vi "NIST Read Binary Data.vi"(0 "Wave File Path IN":path, 5 "error in (no error)":errorcluster, 6 "NIST File Header":T1) -> (14 "Wave File Path OUT":path, 16 "Data":waveform(dbl)[](array[waveform]), 19 "error out":errorcluster)   [LabVIEW 2022 SP3, in "WaveFile.lvclass"]
uses:
  WaveFile.lvclass
  utils/NIST File Header.ctl
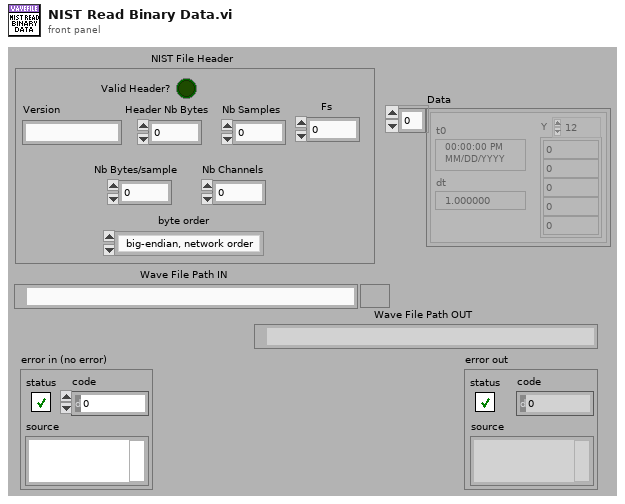
[diagram p1: front panel]
types:
  T1 = typedef "WaveFile.lvclass/NIST File Header.ctl" = cluster{"Version":string, "Header Nb Bytes":i32, "Nb Samples":i32, "Nb Bytes/sample":i32, "Nb Channels":i32, "byte order":enum16{"big-endian, network order", "native, host order", "little-endian"}, "Fs":dbl, "Valid Header?":bool}
  T2 = enum16{"big-endian, network order", "native, host order", "little-endian"}
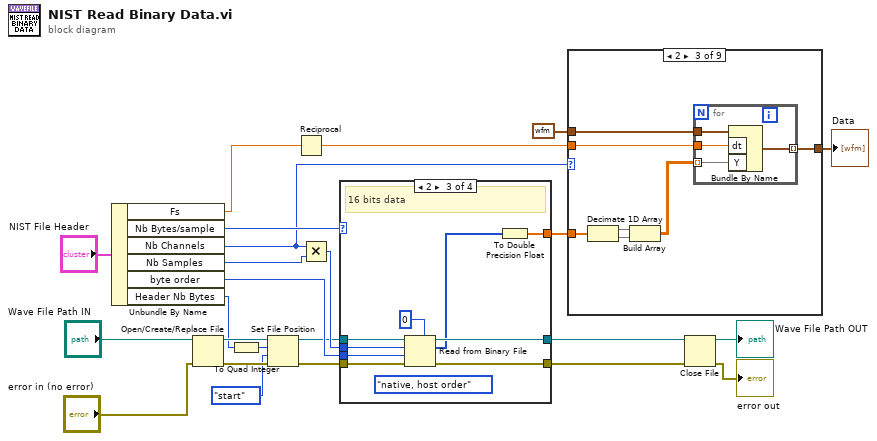
[diagram p0: block diagram]
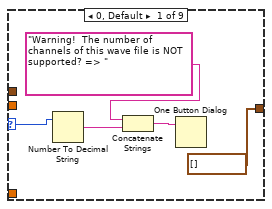
[diagram p2: hidden frame]
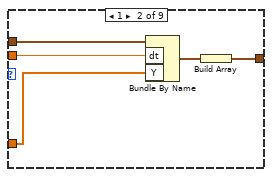
[diagram p3: hidden frame]
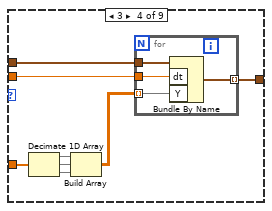
[diagram p4: hidden frame]
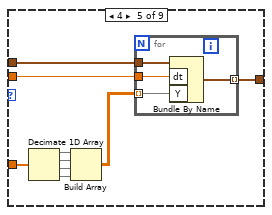
[diagram p5: hidden frame]
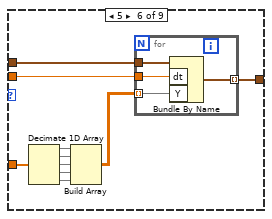
[diagram p6: hidden frame]
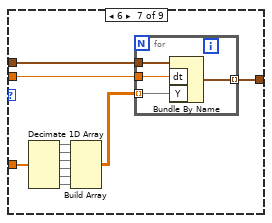
[diagram p7: hidden frame]
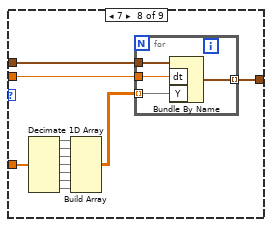
[diagram p8: hidden frame]
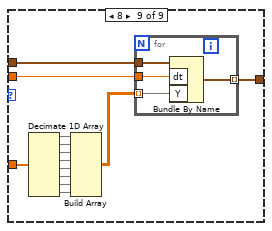
[diagram p9: hidden frame]
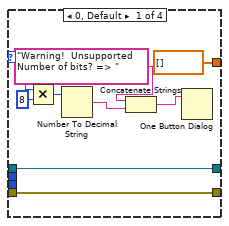
[diagram p10: hidden frame]
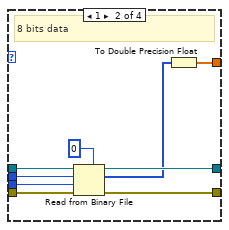
[diagram p11: hidden frame]
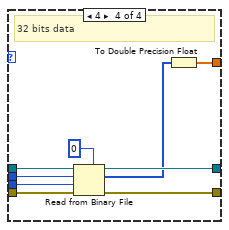
[diagram p12: hidden frame]
diagram:
  n1 = Unbundle By Name("NIST File Header") -> ("Fs"=w14:dbl, "Nb Bytes/sample"=w18:i32, "Nb Channels"=w15:i32, "Nb Samples"=w17:i32, "byte order"=w23:T2, "Header Nb Bytes"=w3:i32)
  n2 = Open/Create/Replace File(file path (use dialog)="Wave File Path IN", error in="error in (no error)") -> (refnum out=w7:refnum<file>, error out=w4:errorcluster)  [unwired: 4 in, 1 out]
  n3 = To Quad Integer(1:w3) -> (0:w2:i64)
  n4 = Set File Position(offset (in bytes) (0)=w2, refnum=w7, from (0:start)=enum16{"start", "end", "current"}."start", error in=w4) -> (refnum out=w6:refnum<file>, error out=w5:errorcluster)
  n5 = Reciprocal(x=w14) -> (1/x=w13:dbl)
  n6 = Multiply(x=w15, y=w17) -> (x*y=w16:i32)
  n7 = case shown="2" w18 {
    selector: w18 -> [w30 _ _ _]
    tunnel: w6 -> [w32 w42 w51 w60]
    tunnel: w5 -> [w31 w41 w50 w59]
    tunnel: w23 -> [_ w34 w43 w58]
    tunnel: w16 -> [_ w40 w49 w57]
    tunnel: [w32 w39 w48 w56] -> w20
    tunnel: [w31 w38 w47 w55] -> w19
    tunnel: [dbl[] [] w35 w44 w52] -> w11
    frame 0, Default {
      n8 = Multiply(x=w30, y=8) -> (x*y=w28:i32)
      n9 = Number To Decimal String(number=w28) -> (decimal integer string=w26:string)  [unwired: 1 in]
      n10 = Concatenate Strings("Warning!  Unsupported Number of bits? => " ("message"), w26) -> (w25:string)
      n11 = One Button Dialog(message=w25) -> ()  [unwired: 1 in, 1 out]
    }
    frame 1 {
      # "8 bits data"
      n12 = Read from Binary File(5:i8 0, 8:w41, 9:w34, 10:w40, 11:w42) -> (0:w38:errorcluster, 2:w36:i8[], 3:w39:refnum<file>)  [unwired: 1 in, 1 out]
      n13 = To Double Precision Float(number=w36) -> (double precision float=w35:dbl[])
    }
    frame 2 {
      (unwired) T2."native, host order" ("byte order (0:big-endian, network order)")
      # "16 bits data"
      n14 = Read from Binary File(5:i16 0, 8:w50, 9:w43, 10:w49, 11:w51) -> (0:w47:errorcluster, 2:w45:i16[], 3:w48:refnum<file>)  [unwired: 1 in, 1 out]
      n15 = To Double Precision Float(number=w45) -> (double precision float=w44:dbl[])
    }
    frame 4 {
      # "32 bits data"
      n16 = Read from Binary File(5:0, 8:w59, 9:w58, 10:w57, 11:w60) -> (0:w55:errorcluster, 2:w53:i32[], 3:w56:refnum<file>)  [unwired: 1 in, 1 out]
      n17 = To Double Precision Float(number=w53) -> (double precision float=w52:dbl[])
    }
  }
  n18 = case shown="2" w15 {
    selector: w15 -> [w63 _ _ _ _ _ _ _ _]
    tunnel: w13 -> [_ w70 w77 w89 w102 w116 w131 w147 w164]
    tunnel: waveform(dbl) {"t0"=timestamp(0 s since 1904-01-01), "dt"=1.0, "Y"=[]} ("waveform") -> [_ w69 w76 w88 w101 w115 w130 w146 w163]
    tunnel: w11 -> [_ w68 w75 w87 w100 w114 w129 w145 w162]
    tunnel: [waveform(dbl)[] [] w66 w71 w83 w96 w110 w125 w141 w158] -> w10
    frame 0, Default {
      n19 = Number To Decimal String(number=w63) -> (decimal integer string=w64:string)  [unwired: 1 in]
      n20 = Concatenate Strings("Warning!  The number of channels of this wave file is NOT supported? => " ("message"), w64) -> (w61:string)
      n21 = One Button Dialog(message=w61) -> ()  [unwired: 1 in, 1 out]
    }
    frame 1 {
      n22 = Bundle By Name(cluster=w69, "dt"=w70, "Y"=w68) -> (w67:waveform(dbl))
      n23 = Build Array(w67) -> (w66:waveform(dbl)[])
    }
    frame 2 {
      n24 = Decimate 1D Array(w75) -> (w74:dbl[], w73:dbl[])
      n25 = Build Array(w74, w73) -> (w72:dbl[][])
      n26 = for {
        tunnel: w77 -> [w81]
        tunnel: w76 -> [w80]
        tunnel: w72 -> [w79] mode=indexing
        tunnel: [w78] -> w71 mode=indexing
        n27 = Bundle By Name(cluster=w80, "dt"=w81, "Y"=w79) -> (w78:waveform(dbl))
      }
    }
    frame 3 {
      n28 = Decimate 1D Array(w87) -> (w86:dbl[], w85:dbl[], w82:dbl[])
      n29 = Build Array(w86, w85, w82) -> (w84:dbl[][])
      n30 = for {
        tunnel: w89 -> [w93]
        tunnel: w88 -> [w92]
        tunnel: w84 -> [w91] mode=indexing
        tunnel: [w90] -> w83 mode=indexing
        n31 = Bundle By Name(cluster=w92, "dt"=w93, "Y"=w91) -> (w90:waveform(dbl))
      }
    }
    frame 4 {
      n32 = Decimate 1D Array(w100) -> (w99:dbl[], w98:dbl[], w95:dbl[], w94:dbl[])
      n33 = Build Array(w99, w98, w95, w94) -> (w97:dbl[][])
      n34 = for {
        tunnel: w102 -> [w106]
        tunnel: w101 -> [w105]
        tunnel: w97 -> [w104] mode=indexing
        tunnel: [w103] -> w96 mode=indexing
        n35 = Bundle By Name(cluster=w105, "dt"=w106, "Y"=w104) -> (w103:waveform(dbl))
      }
    }
    frame 5 {
      n36 = Decimate 1D Array(w114) -> (w113:dbl[], w112:dbl[], w109:dbl[], w108:dbl[], w107:dbl[])
      n37 = Build Array(w113, w112, w109, w108, w107) -> (w111:dbl[][])
      n38 = for {
        tunnel: w116 -> [w120]
        tunnel: w115 -> [w119]
        tunnel: w111 -> [w118] mode=indexing
        tunnel: [w117] -> w110 mode=indexing
        n39 = Bundle By Name(cluster=w119, "dt"=w120, "Y"=w118) -> (w117:waveform(dbl))
      }
    }
    frame 6 {
      n40 = Decimate 1D Array(w129) -> (w128:dbl[], w127:dbl[], w124:dbl[], w123:dbl[], w122:dbl[], w121:dbl[])
      n41 = Build Array(w128, w127, w124, w123, w122, w121) -> (w126:dbl[][])
      n42 = for {
        tunnel: w131 -> [w135]
        tunnel: w130 -> [w134]
        tunnel: w126 -> [w133] mode=indexing
        tunnel: [w132] -> w125 mode=indexing
        n43 = Bundle By Name(cluster=w134, "dt"=w135, "Y"=w133) -> (w132:waveform(dbl))
      }
    }
    frame 7 {
      n44 = Decimate 1D Array(w145) -> (w144:dbl[], w143:dbl[], w140:dbl[], w139:dbl[], w138:dbl[], w137:dbl[], w136:dbl[])
      n45 = Build Array(w144, w143, w140, w139, w138, w137, w136) -> (w142:dbl[][])
      n46 = for {
        tunnel: w147 -> [w151]
        tunnel: w146 -> [w150]
        tunnel: w142 -> [w149] mode=indexing
        tunnel: [w148] -> w141 mode=indexing
        n47 = Bundle By Name(cluster=w150, "dt"=w151, "Y"=w149) -> (w148:waveform(dbl))
      }
    }
    frame 8 {
      n48 = Decimate 1D Array(w162) -> (w161:dbl[], w160:dbl[], w157:dbl[], w156:dbl[], w155:dbl[], w154:dbl[], w153:dbl[], w152:dbl[])
      n49 = Build Array(w161, w160, w157, w156, w155, w154, w153, w152) -> (w159:dbl[][])
      n50 = for {
        tunnel: w164 -> [w168]
        tunnel: w163 -> [w167]
        tunnel: w159 -> [w166] mode=indexing
        tunnel: [w165] -> w158 mode=indexing
        n51 = Bundle By Name(cluster=w167, "dt"=w168, "Y"=w166) -> (w165:waveform(dbl))
      }
    }
  }
  "Data" <- w10
  n52 = Close File(refnum=w20, error in=w19) -> (path=→"Wave File Path OUT":path, error out=→"error out":errorcluster)
